vi "PH_ImageOperator.Energy Calculation.vi"(0 "i ref in":refnum<vi>, 5 "error in (no error)":errorcluster) -> (14 "i ref out":refnum<vi>, 19 "error out":errorcluster)   [LabVIEW 2014, in "PH_ImageOperator.lvlib"]
doc: "This VI includes everything related to energy calculation and indicating."
uses:
  PH_ImageOperator.lvlib
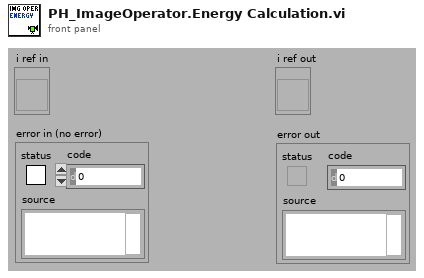
[diagram p1: front panel]
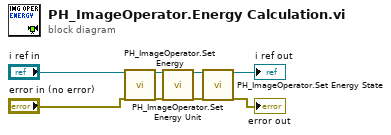
[diagram p0: block diagram]
diagram:
  n1 = call "PH_ImageOperator.Set Energy.vi"("i ref in"="i ref in", "error in (no error)"="error in (no error)") -> ("i ref out"=w3:refnum<vi>, "error out"=w1:errorcluster)  [unwired: 16 in]
  n2 = call "PH_ImageOperator.Set Energy Unit.vi"("i ref in"=w3, "error in (no error)"=w1) -> ("i ref out"=w4:refnum<vi>, "error out"=w2:errorcluster)  [unwired: 16 in]
  n3 = call "PH_ImageOperator.Set Energy State.vi"("i ref in"=w4, "error in (no error)"=w2) -> ("i ref out"=→"i ref out":refnum<vi>, "error out"=→"error out":errorcluster)  [unwired: 16 in]
